vi "Theta2ROV (SubVI).vi"(8 "omega_mti":dbl[](array[numeric])=[0.0, 0.0, 0.0], 9 "MTi_Theta_off":dbl[](array[numeric])=[0.0, 0.0, 0.0], 10 "THETA_hat":dbl[](array[numeric])=[0.0, 0.0, 0.0], 11 "omega_hat":dbl[](array[numeric])=[0.0, 0.0, 0.0]) -> (0 "omega_rov_non_filtered":dbl[](array[numeric]), 2 "THETA_rov":dbl[](array[numeric]), 3 "omega_rov":dbl[](array[numeric]))   [LabVIEW 2014, in "Observer Library.lvlib" / "Attitude Observer.lvclass"]
uses:
  Attitude Observer.lvclass
  <vilib>/imath/engines/lvmath2/RunTimeEngine/IndexRead/NIMS V(S).vi
  <instcachedir>/0/NIMS V(S)_0488751826AF41519A22953C041130DC.lvgen/NIMS V(S)_0488751826AF41519A22953C041130DC_000.vi
  <vilib>/imathl/engines/lvmath/Functions/Error Handling/Create Error.vi
  <vilib>/imath/engines/lvmath2/RunTimeEngine/ArithmeticOperatorToken/NIMS_ArithmeticOperator_multmx(M,CV).vi
  <instcachedir>/0/NIMS_ArithmeticOperator_multmx(M,CV)_787B4652E60B4C52835A7FB23671E425.lvgen/NIMS_ArithmeticOperator_multmx(M,CV)_787B4652E60B4C52835A7FB23671E425_000.vi
  <vilib>/imath/engines/lvmath2/RunTimeEngine/ArithmeticOperatorToken/NIMS_ArithmeticOperator_multmx-internal.vi
  <instcachedir>/0/NIMS_ArithmeticOperator_multmx-internal_D7C5C88E94B94895A818D3A8E50A4506.lvgen/NIMS_ArithmeticOperator_multmx-internal_D7C5C88E94B94895A818D3A8E50A4506_004.vi
  <vilib>/imath/engines/lvmath2/RunTimeEngine/ErrorHandling/NIMS_Create Error From Enums.vi
  <vilib>/imath/engines/lvmath2/RunTimeEngine/NodeEndStatement/NIMS_NodeEndStatement_Get Vector.vi
  <instcachedir>/0/NIMS_NodeEndStatement_Get Vector_00D1625602D843AD9D7EC134A9EC13A2.lvgen/NIMS_NodeEndStatement_Get Vector_00D1625602D843AD9D7EC134A9EC13A2_001.vi
  <vilib>/imath/engines/lvmath/Functions/Error Handling/MergeErrorsWrapper.vi
  <vilib>/imath/engines/lvmath2/RunTimeEngine/NodeEndStatement/NIMS_NodeEndStatement_Output.vi
  <instcachedir>/0/NIMS_NodeEndStatement_Output_53EC0D466D134D7ABD903AC30B43404B.lvgen/NIMS_NodeEndStatement_Output_53EC0D466D134D7ABD903AC30B43404B_005.vi
  <vilib>/imath/engines/lvmath2/RunTimeEngine/ErrorHandling/NIMS_Finalize Error.vi
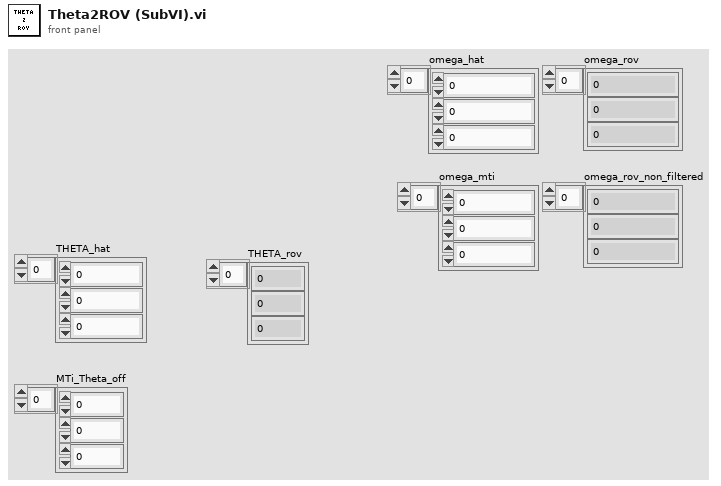
[diagram p1: front panel]
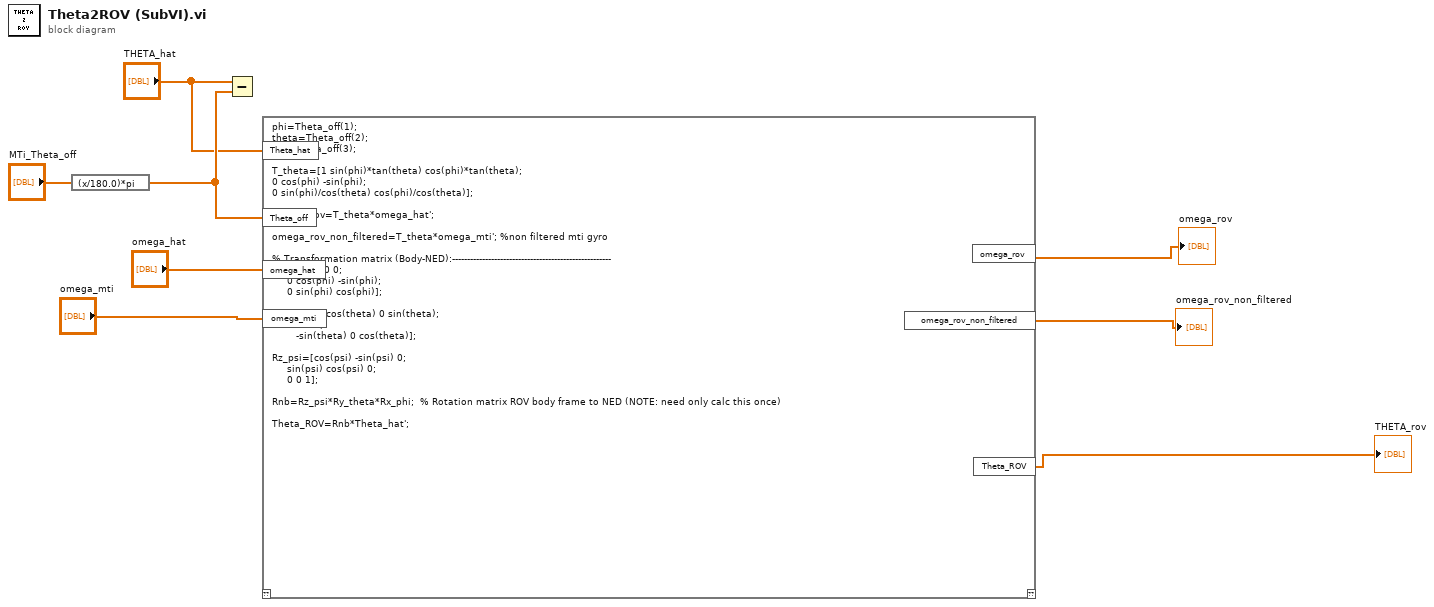
[diagram p0: block diagram]
diagram:
  n1 = expression code="(x/180.0)*pi" ("degrees to radians")("MTi_Theta_off") -> (w3:dbl[])
  n2 = Subtract(x="THETA_hat", y=w3) -> ()  [unwired: 1 out]
  n3 = mathscript code="phi=Theta_off(1);\ntheta=Theta_off(2);\npsi=Theta_off(3);\n\nT_theta=[1 sin(phi)*tan(theta) cos(phi)*tan(theta);\n0 cos(phi) -sin(phi);\n0 sin(phi)/cos(theta) cos(phi)/cos(theta)];\n\nomega_rov=T_theta*omega_hat';\n\nomega_rov_non_filtered=T_theta*omega_mti'; %non filtered mti gyro\n\n% Transformation matrix (Body-NED):-----------------------------------------------------\nRx_phi=[1 0 0;\n     0 cos(phi) -sin(phi);\n     0 sin(phi) cos(phi)];\n\nRy_theta=[cos(theta) 0 sin(theta);\n        0 1 0;\n        -sin(theta) 0 cos(theta)];\n \nRz_psi=[cos(psi) -sin(psi) 0;\n     sin(psi) cos(psi) 0;\n     0 0 1]; \n \nRnb=Rz_psi*Ry_theta*Rx_phi;  % Rotation matrix ROV body frame to NED (NOTE: need only calc this once)\n\nTheta_ROV=Rnb*Theta_hat';"("Theta_off"=w3, "omega_hat"="omega_hat", "omega_mti"="omega_mti", "Theta_hat"="THETA_hat") -> ("omega_rov"=→"omega_rov":dbl[], "omega_rov_non_filtered"=→"omega_rov_non_filtered":dbl[], "Theta_ROV"=→"THETA_rov":dbl[])  [unwired: 1 in, 1 out]
